vi "areaCalculation.vi"(8 "error in (no error)":errorcluster, 9 "filteredSignal":dbl[](array[numeric]), 10 "Duration":dbl[](array[numeric]), 11 "iValesLocation(Samples)":dbl[](array[numeric])) -> (0 "error out":errorcluster, 1 "meanArea/numOsci":dbl, 2 "meanArea":dbl format="%.2f")   [LabVIEW 2012]
uses:
  <vilib>/Analysis/baseanly.llb/Mean (DBL).vi
  <vilib>/Analysis/NI_AALBase.lvlib
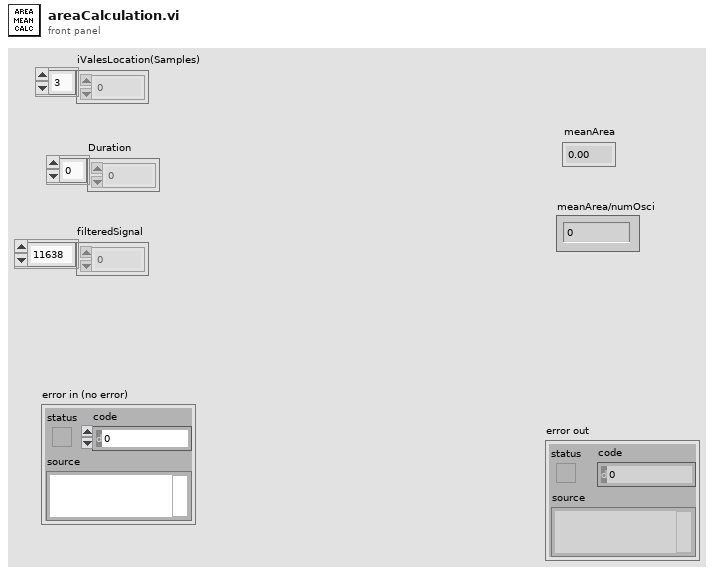
[diagram p1: front panel]
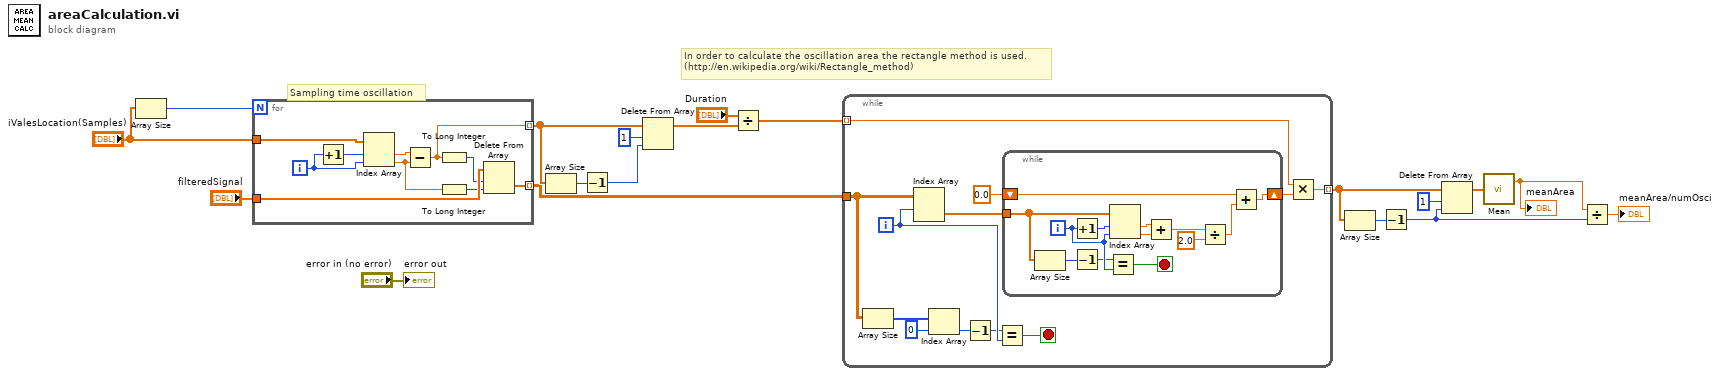
[diagram p0: block diagram]
diagram:
  # "In order to calculate the oscillation area the rectangle method is used.\n(http://en.wikipedia.org/wiki/Rectangle_method)"
  # "Sampling time oscillation"
  n1 = Array Size(array="iValesLocation(Samples)") -> (size(s)=w15:i32)
  n2 = for {
    N: w15 -> [_]
    tunnel: "iValesLocation(Samples)" -> [w29]
    tunnel: [w20] -> w18 mode=indexing
    tunnel: "filteredSignal" -> [w26]
    tunnel: [w21] -> w8 mode=indexing
    i -> [w28]
    n3 = Increment(x=w28) -> (x+1=w27:i32)
    n4 = Index Array(array=w29, index #1=w27, index #2=w28) -> (element #1=w24:dbl, element #2=w25:dbl)
    n5 = Subtract(x=w24, y=w25) -> (x-y=w20:dbl)
    n6 = To Long Integer(number=w20) -> (32bit integer=w23:i32)
    n7 = To Long Integer(number=w25) -> (32bit integer=w22:i32)
    n8 = Delete From Array(array=w26, length=w23, index=w22) -> (deleted portion=w21:dbl[])  [unwired: 1 out]
  }
  n9 = Array Size(array=w18) -> (size(s)=w17:i32)
  n10 = Decrement(x=w17) -> (x-1=w13:i32)
  n11 = Delete From Array(array=w18, length=1, index=w13) -> (array with subset deleted=w11:dbl[])  [unwired: 1 out]
  n12 = Divide(x="Duration", y=w11) -> (x/y=w10:dbl[])
  n13 = while {
    tunnel: w10 -> [w31] mode=indexing
    tunnel: w8 -> [w38]
    tunnel: [w33] -> w7 mode=indexing
    i -> [w39]
    stop <- w41 stop-if-true
    n14 = Array Size(array=w38) -> (size(s)=w37:i32[])
    n15 = Index Array(array=w38, index (row)=w39) -> (element=w30:dbl[])  [unwired: 1 in]
    n16 = Index Array(array=w37, index=0) -> (element=w35:i32)
    n17 = Decrement(x=w35) -> (x-1=w34:i32)
    n18 = Equal?(x=w34, y=w39) -> (x = y?=w41:bool)
    n19 = while {
      tunnel: w30 -> [w54]
      shift-right: [w46] -> w32
      shift-left: 0.0 -> [w45]
      i -> [w50]
      stop <- w52 stop-if-true
      n20 = Array Size(array=w54) -> (size(s)=w53:i32)
      n21 = Increment(x=w50) -> (x+1=w51:i32)
      n22 = Decrement(x=w53) -> (x-1=w44:i32)
      n23 = Equal?(x=w44, y=w50) -> (x = y?=w52:bool)
      n24 = Index Array(array=w54, index #1=w51, index #2=w50) -> (element #1=w49:dbl, element #2=w48:dbl)
      n25 = Add(x=w49, y=w48) -> (x+y=w43:dbl)
      n26 = Divide(x=w43, y=2.0) -> (x/y=w42:dbl)
      n27 = Add(x=w45, y=w42) -> (x+y=w46:dbl)
    }
    n28 = Multiply(x=w31, y=w32) -> (x*y=w33:dbl)
  }
  n29 = Array Size(array=w7) -> (size(s)=w3:i32)
  n30 = Decrement(x=w3) -> (x-1=w2:i32)
  n31 = Delete From Array(array=w7, length=1, index=w2) -> (array with subset deleted=w5:dbl[])  [unwired: 1 out]
  n32 = call-poly <vilib>:"Mean.vi"("X"=w5) -> ("mean"=w4:dbl)  [unwired: 1 out]
  "meanArea" <- w4
  n33 = Divide(x=w4, y=w2) -> (x/y=→"meanArea/numOsci":dbl)
  "error out" <- "error in (no error)"
